vi "Check For Empty Path.vi"(8 "Error In":errorcluster, 11 "Upload Type":u16) -> (0 "Error Out":errorcluster, 1 "Good Paths?":bool=TRUE, 2 "Arduino Base Path":path, 3 "Firmware Builds Base Path":path)   [LabVIEW 2020, in "LMH-LINX.lvlib"]
uses:
  LMH-LINX.lvlib
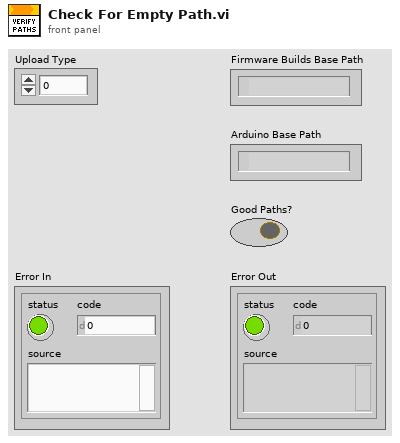
[diagram p1: front panel]
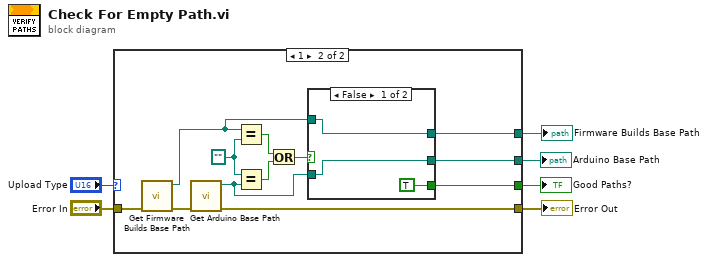
[diagram p0: block diagram]
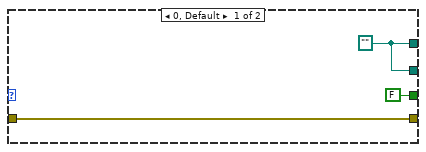
[diagram p2: hidden frame]
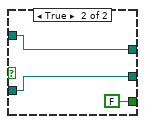
[diagram p3: hidden frame]
diagram:
  n1 = case shown="1" "Upload Type" {
    tunnel: "Error In" -> [w9 w17]
    tunnel: [w9 w15] -> w4
    tunnel: [w8 w12] -> w3
    tunnel: [w8 w11] -> w2
    tunnel: [FALSE w10] -> w1
    frame 0, Default {
      w8 = path ""
    }
    frame 1 {
      w19 = path ""
      n2 = call "Get Firmware Builds Base Path.vi"("Error In"=w17) -> ("Error Out"=w16:errorcluster, "Firmware Builds Base Path"=w14:path)  [unwired: 9 in]
      n3 = call "Get Arduino Base Path.vi"("Error In"=w16) -> ("Error Out"=w15:errorcluster, "Arduino Base Path"=w13:path)  [unwired: 9 in]
      n4 = Equal?(x=w14, y=w19) -> (x = y?=w20:bool)
      n5 = Equal?(x=w19, y=w13) -> (x = y?=w21:bool)
      n6 = Or(x=w20, y=w21) -> (x .or. y?=w18:bool)
      n7 = case shown="False" w18 {
        tunnel: w14 -> [w24 w26]
        tunnel: w13 -> [w23 w25]
        tunnel: [w24 w26] -> w12
        tunnel: [w23 w25] -> w11
        tunnel: [TRUE FALSE] -> w10
        frame False {
        }
        frame True {
        }
      }
    }
  }
  "Error Out" <- w4
  "Firmware Builds Base Path" <- w3
  "Arduino Base Path" <- w2
  "Good Paths?" <- w1
